vi "Reset Control.vi"(0 "GEA2 Reference In":refnum<k24>, 11 "Error In":errorcluster) -> (4 "GEA2 Reference Out":refnum<k24>, 6 "Pass/Fail?":bool, 8 "Report Text":string, 15 "Error Out":errorcluster)   [LabVIEW 2018, in "2015 VA Washer.lvlib"]
doc: "Use this VI to reset the board."
uses:
  Projects/2015 VA Washer.lvlib
  D:/Common/LabVIEW GEA2 Toolkit/source/GEA3 DLL Source/GeaCommunication.dll
  Common/LabVIEW GEA2 Toolkit/source/GEA3 DLL Source/GeaCommunication.dll
  Common/LabVIEW GEA2 Toolkit/GEA3/type defs/ERD Write Data In.ctl
  Common/LabVIEW GEA2 Toolkit/GEA3/type defs/Data Type.ctl
  Common/LabVIEW GEA2 Toolkit/GEA3/type defs/Source_Destination.ctl
  C:/Users/iallatyp/Desktop/New folder/GEA3/library/GEA2_Toolkit.lvlib
panel:
  out "Time to fault code clear":dbl
  out "Time to fault code set (s)":dbl
  in  "Standalone?":bool
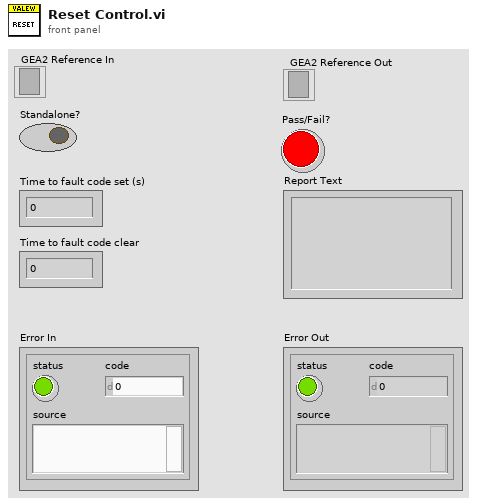
[diagram p1: front panel]
types:
  T1 = typedef "GEA2_Toolkit.lvlib/Source_Destination.ctl" = cluster{"Source":u8, "Destination":u8}
  T2 = typedef "GEA2_Toolkit.lvlib/ERD Write Data In.ctl" = cluster{"ERD Number":u16, "Data Type":T3, "Data":string}
  T3 = typedef "GEA2_Toolkit.lvlib/Data Type.ctl" = enum16{"string", "boolean", "uint8_t", "uint16_t", "uint32_t", "uint64_t", "int8_t", "int16_t", "int32_t", "int64_t"}
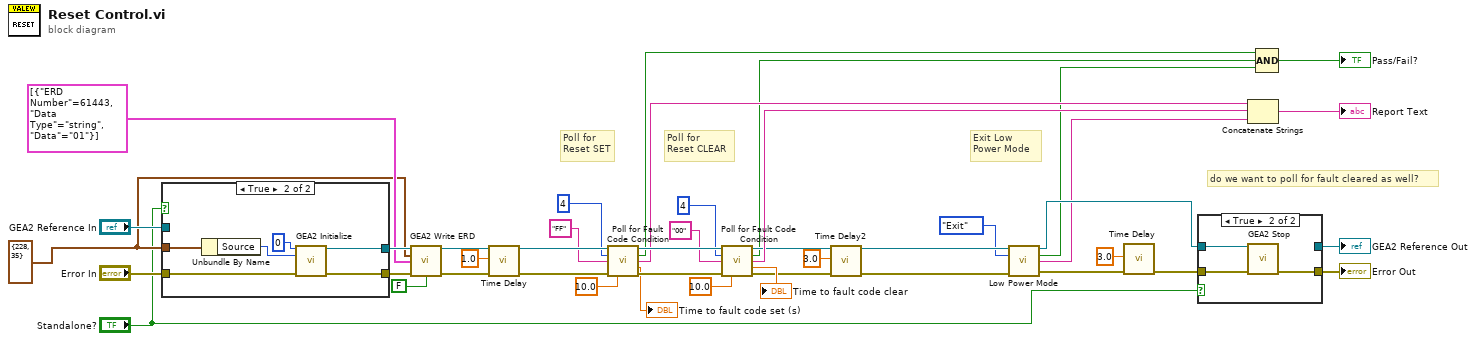
[diagram p0: block diagram]
diagram:
  w29 = T1 {"Source"=228, "Destination"=35} ("GEA Inputs")
  # "Exit Low \nPower Mode"
  # "Poll for\nReset CLEAR"
  # "Poll for\nReset SET"
  # "do we want to poll for fault cleared as well?"
  n1 = case shown="True" "Standalone?" {
    tunnel: "Error In" -> [w42 w49]
    tunnel: [w42 w48] -> w36
    tunnel: "GEA2 Reference In" -> [w43 _]
    tunnel: [w43 w47] -> w41
    tunnel: w29 -> [_ w45]
    frame False {
    }
    frame True {
      n2 = Unbundle By Name(w45) -> ("Source"=w46:u8)
      n3 = call "GEA2 Initialize.vi"("Board Index"=0, "Source Address"=w46, "error in"=w49) -> ("GEA2 Reference Out"=w47:refnum<k24>, "error out"=w48:errorcluster)  [unwired: 10 in, 1 out]
    }
  }
  n4 = call "GEA2 Write ERD.vi"("GEA2 Reference In"=w41, "GEA Inputs"=w29, "Write ERD List"=T2[] [{"ERD Number"=61443, "Data Type"=enum."string", "Data"="01"}], "Error In"=w36, "Verify ERD Response?"=FALSE) -> ("GEA2 Reference Out"=w34:refnum<k24>, "Error Out"=w12:errorcluster)  [unwired: 8 in, 1 out]
  n5 = call "Time Delay"("error in (no error)"=w12, "Delay Time (s)"=1.0) -> ("error out"=w8:errorcluster)  [unwired: 9 in]
  n6 = call "Poll for Fault Code Condition.vi"("GEA2 Reference In"=w34, "Fault ID (Decimal)"=u16 4, "Fault Status (00/FF)"="FF", "Error In"=w8, "Timeout (s)"=10.0) -> ("GEA2 Reference Out"=w30:refnum<k24>, "Pass/Fail?"=w20:bool, "Report Text"=w26:string, "Time to fault code set (s)"=→"Time to fault code set (s)":dbl, "Error Out"=w31:errorcluster)  [unwired: 6 in]
  n7 = call "Poll for Fault Code Condition.vi"("GEA2 Reference In"=w30, "Fault ID (Decimal)"=u16 4, "Fault Status (00/FF)"="00", "Error In"=w31, "Timeout (s)"=10.0) -> ("GEA2 Reference Out"=w22:refnum<k24>, "Pass/Fail?"=w19:bool, "Report Text"=w25:string, "Time to fault code set (s)"=→"Time to fault code clear":dbl, "Error Out"=w2:errorcluster)  [unwired: 6 in]
  n8 = call "Time Delay2"("error in (no error)"=w2, "Delay Time (s)"=3.0) -> ("error out"=w1:errorcluster)  [unwired: 9 in]
  n9 = call "Low Power Mode.vi"("GEA2 Reference In"=w22, "Action"=enum16{"Enter", "Exit"}."Exit", "Error In"=w1) -> ("GEA2 Reference Out"=w27:refnum<k24>, "Pass/Fail?"=w18:bool, "Report Text"=w24:string, "Error Out"=w5:errorcluster)  [unwired: 9 in]
  n10 = call "Time Delay"("error in (no error)"=w5, "Delay Time (s)"=3.0) -> ("error out"=w4:errorcluster)  [unwired: 9 in]
  n11 = case shown="True" "Standalone?" {
    tunnel: w4 -> [w51 w54]
    tunnel: [w51 w53] -> w40
    tunnel: [w50 _] -> w39
    tunnel: w27 -> [w50 w52]
    frame False {
    }
    frame True {
      n12 = call "GEA2 Stop.vi"("GEA2 Reference In"=w52, "Error In"=w54) -> ("Error Out"=w53:errorcluster)  [unwired: 13 in]
    }
  }
  "Error Out" <- w40
  "GEA2 Reference Out" <- w39
  n13 = Concatenate Strings(w26, w25, w24) -> (→"Report Text":string)
  n14 = Compound Arithmetic op=AND(w20, w19, w18) -> (→"Pass/Fail?":bool)
